vi "Exercise3_week2.vi"() -> ()   [LabVIEW 2015]
panel:
  in  "Numeric 2":dbl
  out "Numeric":dbl
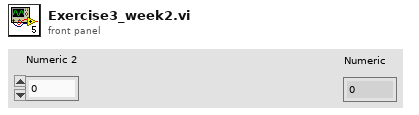
[diagram p1: front panel]
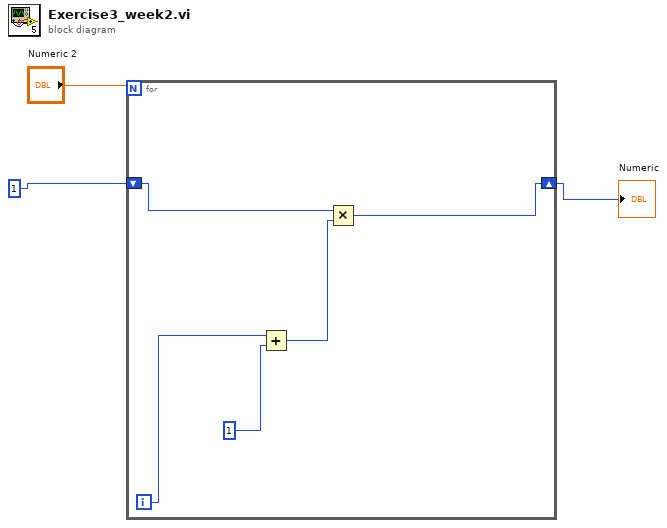
[diagram p0: block diagram]
diagram:
  n1 = for {
    N: "Numeric 2" -> [_]
    shift-right: [w4] -> w2
    shift-left: 1 -> [w5]
    i -> [w7]
    n2 = Add(x=w7, y=1) -> (x+y=w6:i32)
    n3 = Multiply(x=w5, y=w6) -> (x*y=w4:i32)
  }
  "Numeric" <- w2
